vi "Finalize Data.vi"(8 "error in (no error)":errorcluster, 11 "Core Plugins Configuration in":refnum<class "Core Plugins Configuration.lvclass">) -> (0 "error out":errorcluster, 1 "data version":T1, 2 "data":string, 3 "Core Plugins Configuration out":refnum<class "Core Plugins Configuration.lvclass">)   [LabVIEW 2017, in "DSF Core.lvlib" / "Core Plugins Configuration.lvclass"]
uses:
  Core Plugins Configuration.lvclass
  C:/Git/DSF/Core/Classes/Configuration/Configuration.lvclass
  Typedefs/DSF Version Info.ctl
  Core Plugins Configuration.lvclass/Core Plugins Configuration.ctl
  Configuration.lvclass
  DSF Core.lvlib
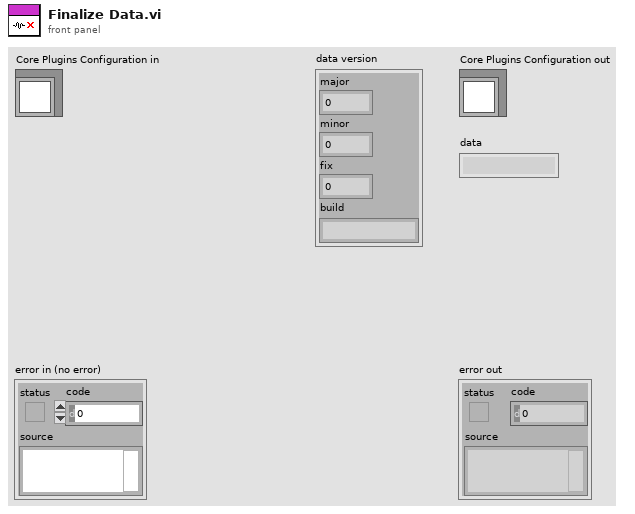
[diagram p1: front panel]
types:
  T1 = typedef "DSF Core.lvlib/DSF Version Info.ctl" = cluster{"major":i32, "minor":i32, "fix":i32, "build":string}
  T2 = typedef "DSF Core.lvlib/Core Plugins Configuration.lvclass/Configuration.ctl" = cluster{"name":string, "components":string[], "cycle timing":T3}
  T3 = typedef "DSF Core.lvlib/DSF Timing Info.ctl" = cluster{"priority":u64, "decimation":u64, "offset":u64}
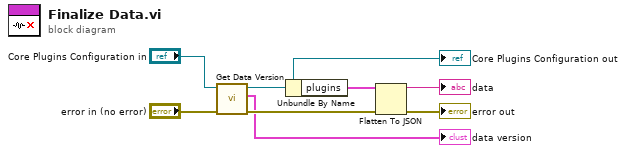
[diagram p0: block diagram]
diagram:
  n1 = call "Get Data Version.vi"("error in (no error)"="error in (no error)", "Configuration in"="Core Plugins Configuration in") -> ("error out"=w7:errorcluster, "data version"=→"data version":T1, "Configuration out"=w2:refnum<class "Core Plugins Configuration.lvclass">)  [unwired: 7 in]
  "Core Plugins Configuration out" <- w2
  n2 = Unbundle By Name(w2) -> ("plugins"=w1:T2[])
  n3 = Flatten To JSON(anything=w1, error in (no error)=w7) -> (JSON string=→"data":string, 11:→"error out":errorcluster)  [unwired: 1 in]
